vi "Commissioning Init.vi"(8 "error in":errorcluster, 11 "SCADA in":refnum<class "EMS.lvclass">) -> (0 "error out":errorcluster, 3 "SCADA out":refnum<class "EMS.lvclass">)   [LabVIEW 2018, in "EMS Core.lvlib" / "EMS.lvclass"]
uses:
  EMS.lvclass
  C:/Program Files (x86)/National Instruments/LabVIEW 2018/vi.lib/ActorFramework/Actor/Actor.lvclass
  Controls/Microgrid State.ctl
  EMS.lvclass/EMS.ctl
  <vilib>/ActorFramework/Message Enqueuer/Message Enqueuer.lvclass/Message Enqueuer.ctl
  <vilib>/ActorFramework/Actor/Actor.lvclass/Actor.ctl
  EMS Messages/Return Microgrid State Msg/Return Microgrid State Msg.lvclass/Return Microgrid State Msg.ctl
  <vilib>/ActorFramework/Message Enqueuer/Enqueue.vi
  <vilib>/ActorFramework/Stop Msg/Stop Msg.lvclass
  C:/Program Files (x86)/National Instruments/LabVIEW 2018/vi.lib/ActorFramework/Message/Message.lvclass
  EMS Messages/Return Microgrid State Msg/Return Microgrid State Msg.lvclass
  <vilib>/ActorFramework/Message Priority Queue/Priority Enqueue.vi
  <vilib>/ActorFramework/Actor/Actor.lvclass
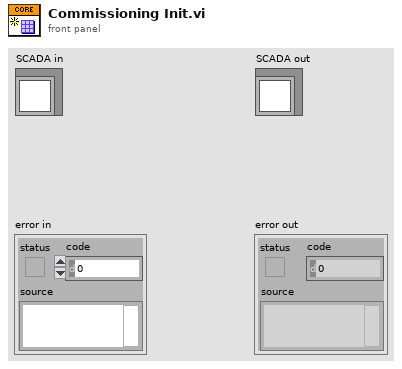
[diagram p1: front panel]
types:
  T1 = typedef "EMS Core.lvlib/EMS.lvclass/Microgrid State.ctl" = enum16{"Discovery", "Commissioning", "Activation", "Blackstart", "OnGrid", "OffGrid", "Island", "Resynchronization", "Manual", "Shutdown", "Stop"}
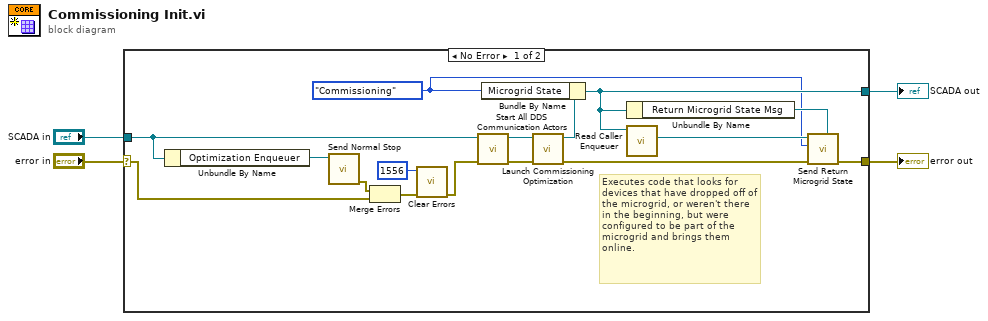
[diagram p0: block diagram]
diagram:
  n1 = case shown="No Error" "error in" {
    selector: "error in" -> [w19 w22]
    tunnel: [w18 w22] -> w3
    tunnel: [w17 w21] -> w1
    tunnel: "SCADA in" -> [w20 w21]
    frame No Error {
      w14 = Microgrid_State."Commissioning" ("Microgrid State")
      # "Executes code that looks for devices that have dropped off of the microgrid, or weren't there in the beginning, but were configured to be part of the microgrid and brings them online."
      n2 = Unbundle By Name(w20) -> ("Optimization Enqueuer"=w11:refnum<class "Message Enqueuer.lvclass">)
      n3 = call <vilib>:"Send Normal Stop.vi"("Message Enqueuer"=w11) -> ("error out"=w8:errorcluster)  [unwired: 10 in]
      n4 = Merge Errors(w8, w19) -> (w7:errorcluster)
      n5 = call <vilib>:"Clear Errors.vi"("error in (no error)"=w7, "specific error code to clear (0: all)"=1556) -> ("error out"=w10:errorcluster)  [unwired: 4 in, 1 out]
      n6 = call "Start All DDS Communication Actors.vi"("error in"=w10, "SCADA in"=w20) -> ("error out"=w13:errorcluster, "SCADA out"=w12:refnum<class "EMS.lvclass">)  [unwired: 8 in]
      n7 = call "Launch Commissioning Optimization.vi"("error in"=w13, "SCADA in"=w12) -> ("error out"=w5:errorcluster, "SCADA out"=w6:refnum<class "EMS.lvclass">)  [unwired: 8 in]
      n8 = Bundle By Name(cluster=w6, "Microgrid State"=w14) -> (w17:refnum<class "EMS.lvclass">)
      n9 = Unbundle By Name(w17) -> ("Return Microgrid State Msg"=w15:refnum<class "Return Microgrid State Msg.lvclass">)
      n10 = call <vilib>:"Read Caller Enqueuer.vi"("Actor"=w17) -> ("Caller Enqueuer"=w16:refnum<class "Message Enqueuer.lvclass">)  [unwired: 10 in]
      n11 = call "Send Return Microgrid State.vi"("Message Type"=w15, "error in (no error)"=w5, "Microgrid State"=w14, "Message Enqueuer"=w16) -> ("error out"=w18:errorcluster)  [unwired: 6 in, 1 out]
    }
    frame Error {
    }
  }
  "error out" <- w3
  "SCADA out" <- w1
